vi "Pi_ColorText.vi"(4 "Bold?":bool, 6 "Color":u32(colorbox), 9 "End":i32=10000, 10 "Start":i32, 11 "String in":refnum<vi>) -> (3 "String out":refnum<vi>)   [LabVIEW 2019]
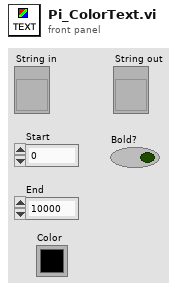
[diagram p1: front panel]
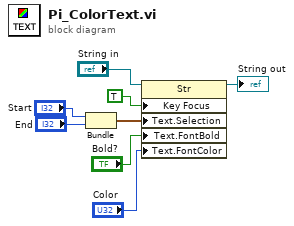
[diagram p0: block diagram]
diagram:
  n1 = Bundle("Start"="Start", "End"="End") -> (w2:cluster{"Start":i32, "End":i32})  [unwired: 1 in]
  n2 = property on="Property Node" class="Str"(reference="String in", "Key Focus"=TRUE, "Text.Selection"=w2, "Text.FontBold"="Bold?", "Text.FontColor"="Color") -> (reference out=→"String out":refnum<vi>)  [unwired: 1 in, 1 out]
